vi "generate xml for slow zstack.vi"(10 "Old File Path":path, 11 "New File Path":path) -> ()   [LabVIEW 2012]
doc: "SciScan 1.2 160622"
uses:
  OME Module/SubVIs/FGV_ExclusionList_Manager_Commands.ctl
  <resource>/objmgr/DOMUserDefRef.rc
  <vilib>/xml/NI_XML.lvlib
panel:
  out "Parse Errors":string
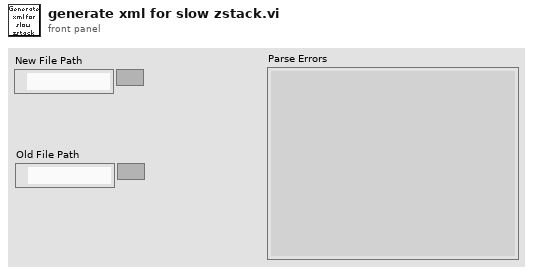
[diagram p1: front panel]
types:
  T1 = typedef "FGV_ExclusionList_Manager_Commands.ctl" = enum16{"Initialize(ReadCSV)", "Get", "CategorizePaths"}
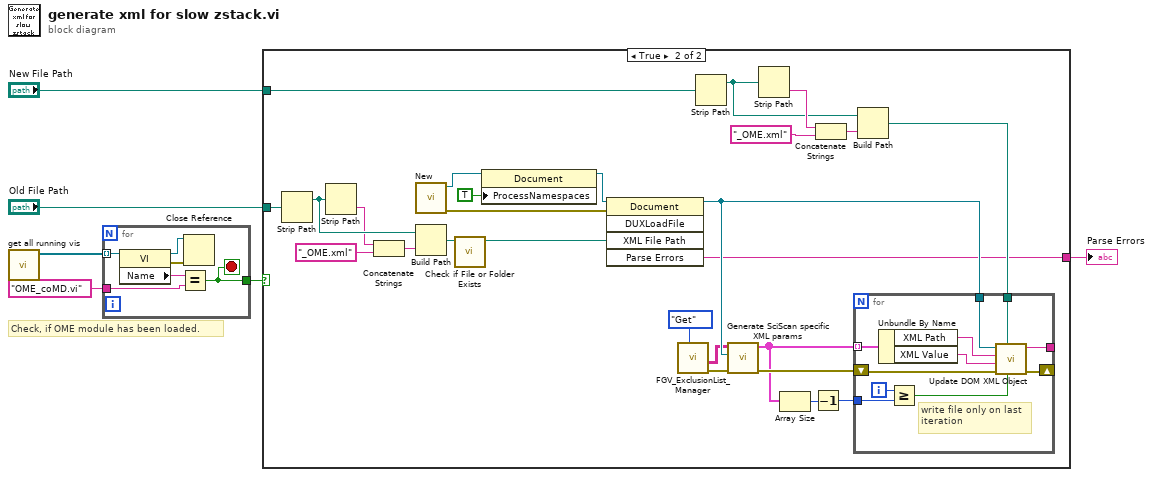
[diagram p0: block diagram]
diagram:
  # "Check, if OME module has been loaded."
  n1 = call "get all running vis.vi"() -> ("RunningVIRefs"=w3:refnum<vi>[])  [unwired: 11 in]
  n2 = for {
    tunnel: w3 -> [w12] mode=indexing
    tunnel: "OME_coMD.vi" ("ItemTag") -> [w9]
    tunnel: [w11] -> w1
    stop <- w11 stop-if-true
    n3 = property class="VI"(reference=w12) -> (reference out=w8:refnum<vi>, error out=w7:errorcluster, "Name"=w10:string)  [unwired: 1 in]
    n4 = Equal?(x=w10, y=w9) -> (x = y?=w11:bool)
    n5 = Close Reference(reference=w8, error in (no error)=w7) -> ()  [unwired: 1 out]
  }
  n6 = case shown="True" w1 {
    tunnel: "New File Path" -> [_ w38]
    tunnel: "Old File Path" -> [_ w32]
    tunnel: [_ w13] -> w4
    frame False {
    }
    frame True {
      n7 = Strip Path(path=w32) -> (stripped path=w36:path)  [unwired: 1 out]
      n8 = Strip Path(path=w36) -> (name=w35:string)  [unwired: 1 out]
      n9 = Concatenate Strings(w35, "_OME.xml" ("string")) -> (w34:string)
      n10 = call <vilib>:"New.vi"() -> ("error out"=w27:errorcluster, "DOM document out"=w29:refnum<k20>)  [unwired: 8 in]
      n11 = Build Path(base path=w36, name or relative path=w34) -> (appended path=w31:path)
      n12 = call <vilib>:"Check if File or Folder Exists.vi"("path"=w31) -> ("dup path"=w37:path)  [unwired: 8 in, 2 out]
      n13 = property class="Document"(reference=w29, "ProcessNamespaces"=TRUE ("Process Namespaces")) -> (reference out=w30:refnum<k20>)  [unwired: 1 in, 1 out]
      n14 = invoke class="Document" method="DUXLoadFile"(reference=w30, error in=w27, "XML File Path"=w37) -> (reference out=w26:refnum<k20>, "Parse Errors"=w13:string)  [unwired: 2 in, 3 out]
      n15 = call "FGV_ExclusionList_Manager.vi"("Actions"=FGV_ExclusionList_Manager_Commands."Get") -> ("error out"=w16:errorcluster, "To Exclude"=w15:string[][])  [unwired: 5 in, 4 out]
      n16 = Strip Path(path=w38) -> (stripped path=w22:path)  [unwired: 1 out]
      n17 = call "Generate SciScan specific XML params.vi"("error in (no error)"=w16, "DOM document IN"=w26, "Non-Tree elements 2D array IN"=w15) -> ("error out"=w20:errorcluster, "Path-Value pairs Array"=w17:cluster{"XML Path":string, "XML Value":string}[])  [unwired: 7 in]
      n18 = Strip Path(path=w22) -> (name=w23:string)  [unwired: 1 out]
      n19 = Array Size(array=w17) -> (size(s)=w18:i32)
      n20 = Decrement(x=w18) -> (x-1=w19:i32)
      n21 = Concatenate Strings(w23, "_OME.xml" ("string")) -> (w24:string)
      n22 = Build Path(base path=w22, name or relative path=w24) -> (appended path=w21:path)
      n23 = for {
        tunnel: w26 -> [w49]
        tunnel: w21 -> [w48]
        tunnel: w17 -> [w43] mode=indexing
        tunnel: w19 -> [w46]
        shift-right: [w40] -> _
        shift-left: w20 -> [w44]
        tunnel: [w39] -> _
        i -> [w47]
        # "write file only on last\niteration"
        n24 = Unbundle By Name(w43) -> ("XML Path"=w42:string, "XML Value"=w41:string)
        n25 = Greater Or Equal?(x=w47, y=w46) -> (x >= y?=w45:bool)
        n26 = call "Update DOM XML Object.vi"("Write to File?"=w45, "XML File Path"=w48, "error in (no error)"=w44, "New Value (String)"=w41, "XPath expression to node"=w42, "DOM Refnum (XML Document)"=w49) -> ("error out"=w40:errorcluster, "XML string out"=w39:string)  [unwired: 4 in]
      }
    }
  }
  "Parse Errors" <- w4
